vi "LoopselFF_1cam.VI"() -> ()   [LabVIEW 2015]
panel:
  out "Signalverlaufgraph":u16[](graph)=[0, 0, 0, 0, 0, 1, 0, 27665, 0, 0, 0, 0, 0, 0, 0, 0, 0, 0, 0, 0, 0, 0, 0, 0, 0, 0, 0, 0, 0, 0, 0, 0, 0, 0, 0, 0, 0, 0, 0, 0, 0, 0, 0, 0, 0, 0, 0, 0, 0, 0, 0, 0, 0, 0, 0, 0, 0, 0, 0, 0, 0, 0, 0, 0, 0, 0, 0, 0, 0, 0, 0, 0, 0, 0, 0, 0, 0, 0, 0, 0, 0, 0, 0, 0, 0, 0, 0, 0, 0, 0, 0, 0, 0, 0, 0, 0, 0, 0, 0, 0, 0, 0, 0, 0, 0, 0, 0, 0, 0, 0, 0, 0, 0, 0, 0, 0, 0, 0, 0, 0, 0, 0, 0, 0, 0, 0, 0, 0, 0, 0, 0, 0, 0, 0, 0, 0, 0, 0, 0, 0, 0, 0, 0, 0, 0, 0, 0, 0, 0, 0, 0, 0, 0, 0, 0, 0, 0, 0, 0, 0, 0, 0, 0, 0, 0, 0, 0, 0, 0, 0, 0, 0, 0, 0, 0, 0, 0, 0, 0, 0, 0, 0, 0, 0, 0, 0, 0, 0, 0, 0, 0, 0, 0, 0, 0, 0, 0, 0, 0, 0, 0, 0, 0, 0, 0, 0, 0, 0, 0, 0, 0, 0, 0, 0, 0, 0, 0, 0, 0, 0, 0, 0, 0, 0, 0, 0, 0, 0, 0, 0, 0, 0, 0, 0, 0, 0, 0, 0, 0, 0, 0, 0, 0, 0, 0, 0, 0, 0, 0, 0, 0, 0, 0, 0, 0, 0, 0, 0, 0, 0, 0, 0, 0, 0, 0, 0, 0, 0, 0, 0, 0, 0, 0, 0, 0, 0, 0, 0, 0, 0, 0, 0, 0, 0, 0, 0, 0, 0, 0, 0, 0, 0, 0, 0, 0, 0, 0, 0, 0, 0, 0, 0, 0, 0, 0, 0, 0, 0, 0, 0, 0, 0, 0, 0, 0, 0, 0, 0, 0, 0, 0, 0, 0, 0, 0, 0, 0, 0, 0, 0, 0, 0, 0, 0, 0, 0, 0, 0, 0, 0, 0, 0, 0, 0, 0, 0, 0, 0, 0, 0, 0, 0, 0, 0, 0, 0, 0, 0, 0, 0, 0, 0, 0, 0, 0, 0, 0, 0, 0, 0, 0, 0, 0, 0, 0, 0, 0, 0, 0, 0, 0, 0, 0, 0, 0, 0, 0, 0, 0, 0, 0, 0, 0, 0, 0, 0, 0, 0, 0, 0, 0, 0, 0, 0, 0, 0, 0, 0, 0, 0, 0, 0, 0, 0, 0, 0, 0, 0, 0, 0, 0, 0, 0, 0, 0, 0, 0, 0, 0, 0, 0, 0, 0, 0, 0, 0, 0, 0, 0, 0, 0, 0, 0, 0, 0, 0, 0, 0, 0, 0, 0, 0, 0, 0, 0, 0, 0, 0, 0, 0, 0, 0, 0, 0, 0, 0, 0, 0, 0, 0, 0, 0, 0, 0, 0, 0, 0, 0, 0, 0, 0, 0, 0, 0, 0, 0, 0, 0, 0, 0, 0, 0, 0, 0, 0, 0, 0, 0, 0, 0, 0, 0, 0, 0, 0, 0, 0, 0, 0, 0, 0, 0, 0, 0, 0, 0, 0, 0, 0, 0, 0, 0, 0, 0, 0, 0, 0, 0, 0, 0, 0, 0, 0, 0, 0, 0, 0, 0, 0, 0, 0, 0, 0, 0, 0, 0, 0, 0, 0, 0, 0, 0, 0, 0, 0, 0, 0, 0, 0, 0, 0, 0, 0, 0, 0, 0, 0, 0, 0, 0, 0, 0, 0, 0, 0, 0, 0, 0, 0, 0, 0, 0, 0, 0, 0, 0, 0, 0, 0, 0, 0, 0, 0, 0, 0, 0, 0, 0, 0, 0, 0, 0, 0, 0, 0, 0, 0, 0, 0, 0, 0, 0, 0, 0, 0, 0, 0, 0, 0, 0, 0, 0, 0, 0, 0, 0, 0, 0, 0, 0, 0, 0, 0, 0, 0, 0, 0, 0, 0, 0, 0, 0, 0, 0, 0, 0, 0, 0, 0, 0, 0, 0, 0, 0, 0, 0, 0, 0, 0, 0, 0, 0, 0, 0, 0, 0, 0, 0, 0, 0, 0, 0, 0, 0, 0, 0, 0, 0, 0, 0, 0, 0, 0, 0, 0, 0, 0, 0, 0, 0, 0, 0, 0, 0, 0, 0, 0, 0, 0, 0, 0, 0, 0, 0, 0, 0, 0, 0, 0, 0, 0, 0, 0, 0, 0, 0, 0, 0, 0, 0, 0, 0, 0, 0, 0, 0, 0, 0, 0, 0, 0, 0, 0, 0, 0, 0, 0, 0, 0, 0, 0, 0, 0, 0, 0, 0, 0, 0, 0, 0, 0, 0, 0, 0, 0, 0, 0, 0, 0, 0, 0, 0, 0, 0, 0, 0, 0, 0, 0, 0, 0, 0, 0, 0, 0, 0, 0, 0, 0, 0, 0, 0, 0, 0, 0, 0, 0, 0, 0, 0, 0, 0, 0, 0, 0, 0, 0, 0, 0, 0, 0, 0, 0, 0, 0, 0, 0, 0, 0, 0, 0, 0, 0, 0, 0, 0, 0, 0, 0, 0, 0, 0, 0, 0, 0, 0, 0, 0, 0, 0, 0, 0, 0, 0, 0, 0, 0, 0, 0, 0, 0, 0, 0, 0, 0, 0, 0, 0, 0, 0, 0, 0, 0, 0, 0, 0, 0, 0, 0, 0, 0, 0, 0, 0, 0, 0, 0, 0, 0, 0, 0, 0, 0, 0, 0, 0, 0, 0, 0, 0, 0, 0, 0, 0, 0, 0, 0, 0, 0, 0, 0, 0, 0, 0, 0, 0, 0, 0, 0, 0, 0, 0, 0, 0, 0, 0, 0, 0, 0, 0, 0, 0, 0, 0, 0, 0, 0, 0, 0, 0, 0, 0, 0, 0, 0, 0, 0, 0, 0, 0, 0, 0, 0, 0, 0, 0, 0, 0, 0, 0, 0, 0, 0, 0, 0, 0, 0, 0, 0, 0, 0, 0, 0, 0, 0, 0, 0, 0, 0, 0, 0, 0, 0, 0, 0, 0, 0, 0, 0, 0, 0, 0, 0, 0, 0, 0, 0, 0, 0, 0, 0, 0, 0, 0, 0, 0, 0, 0, 0, 0, 0, 0, 0, 0, 0, 0, 0, 0, 0, 0, 0, 0, 0, 0, 0, 0, 0, 0, 0, 0, 0, 0, 0, 0, 0, 0, 0, 0, 0, 0, 0, 0, 0, 0, 0, 0, 0, 0, 0, 0, 0, 0, 0, 0, 0, 0, 0, 0, 0, 0, 0, 0, 0, 0, 0, 0, 0, 0, 0, 0, 0, 0, 0, 0, 0, 0, 0, 0, 0, 0, 0, 0, 0, 0, 0, 0, 0, 0, 0, 0, 0, 0, 0, 0, 0, 0, 0, 0, 0, 0, 0, 0, 0, 0, 0, 0, 0, 0]
  in  "Slide":u32(slide)=27666 scale=1.0..60000.0
  in  "stop all":bool
  out "FIFO overflow 2":bool
  in  "extTrig 0/1":u8
  in  "frequency[Hz]":u32
  in  "start new block":bool
  in  "alloc mem":bool
  out "FREE \nRAM MB":u64=14179
  out "BUILT-IN\nRAM MB":u64=16662
  out "SEC":dbl=1.2
  out "MB RAM":u64=125
  in  "pos slope":u8=1
  in  "both slopes":u8
  in  "DAT in 10ns":u32
  in  "no.of samples (nos)":u32=60000
  in  "exposuretime[ms]":dbl=0.02 format="%.3f"
  # "Start with run"
  # "Abort with ESC"
  # "1x"
  # "repeat"
  # "exit here"
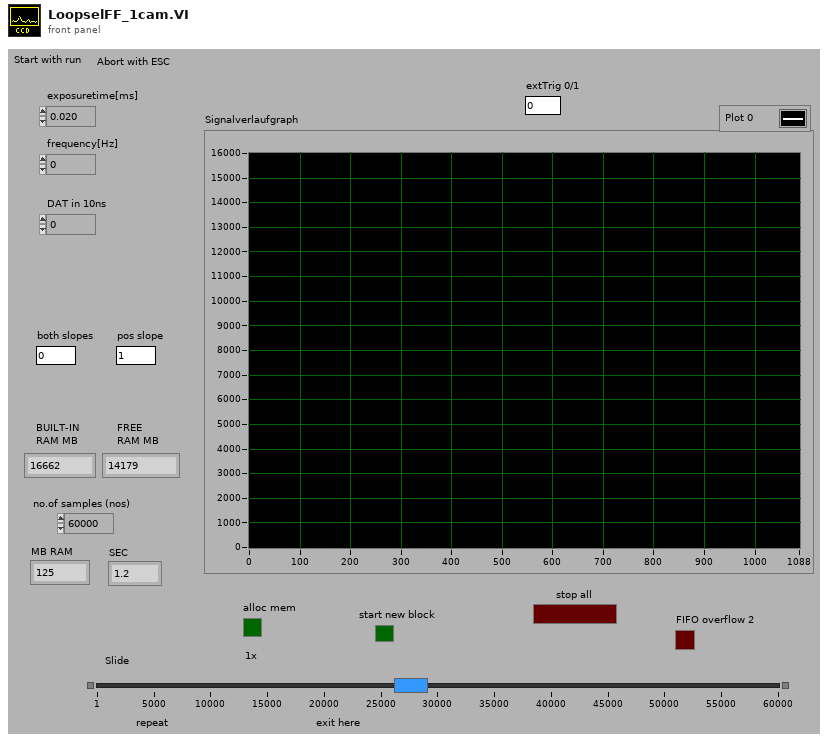
[diagram p1: front panel]
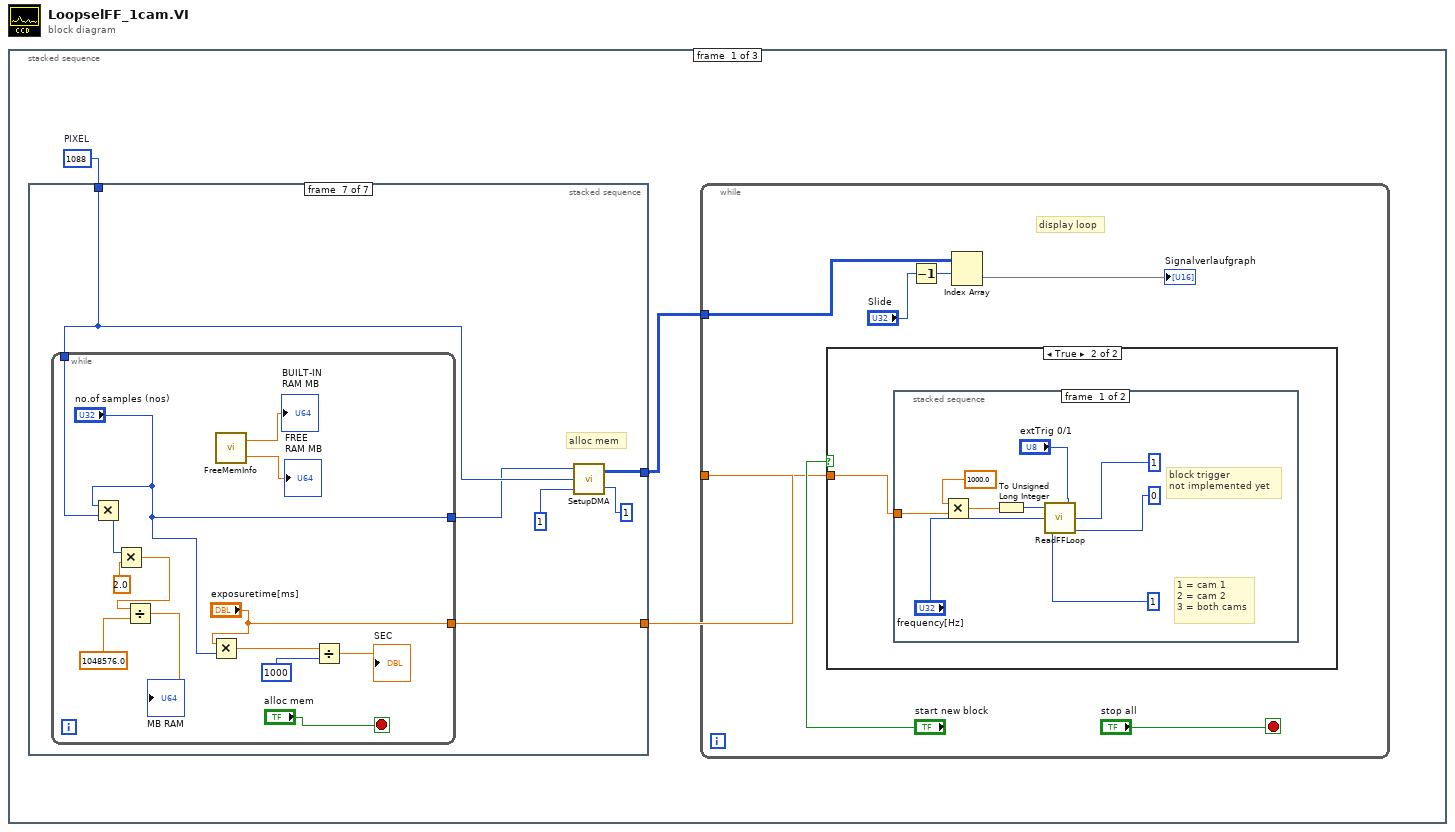
[diagram p0: block diagram]
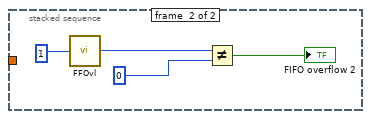
[diagram p3: hidden frame]
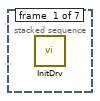
[diagram p4: hidden frame]
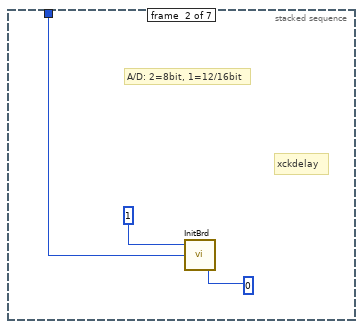
[diagram p5: hidden frame]
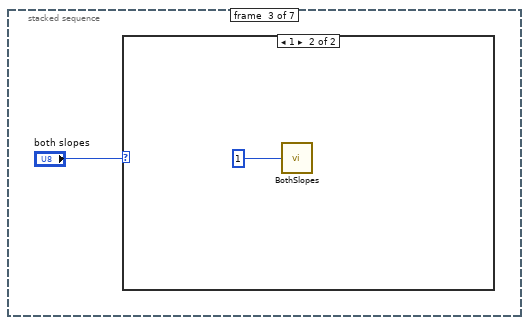
[diagram p6: hidden frame]
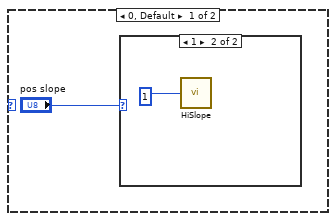
[diagram p7: hidden frame]
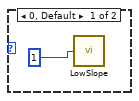
[diagram p8: hidden frame]
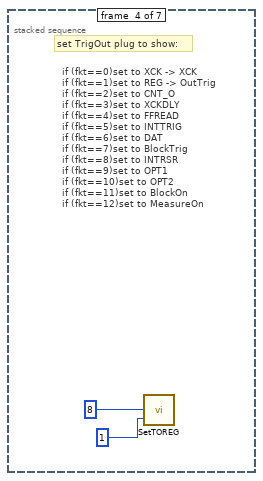
[diagram p9: hidden frame]
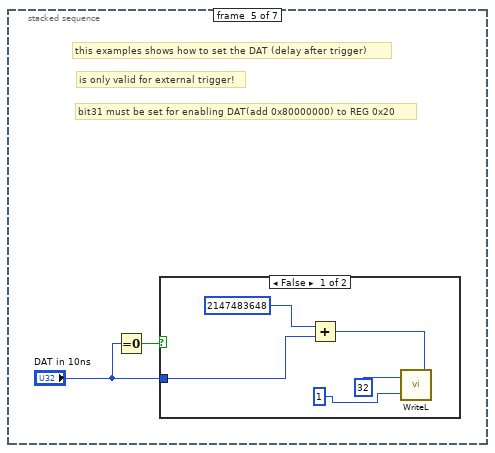
[diagram p10: hidden frame]
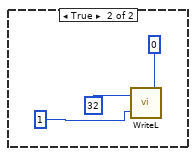
[diagram p11: hidden frame]
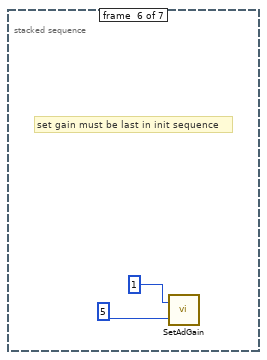
[diagram p12: hidden frame]
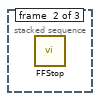
[diagram p13: hidden frame]
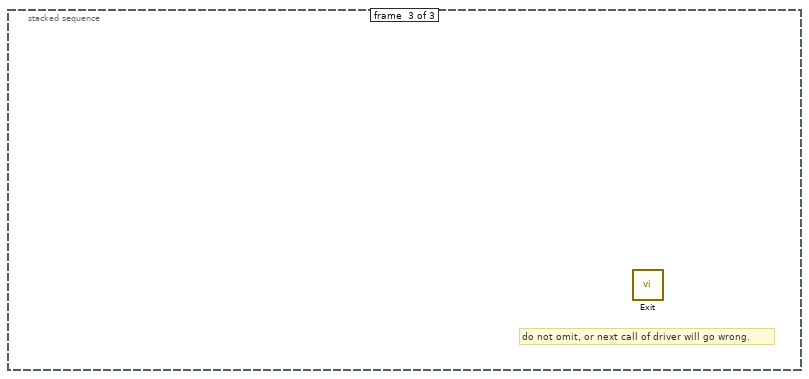
[diagram p14: hidden frame]
diagram:
  n1 = stacked-sequence {
    frame #0 {
      w3 = u32 1088  # PIXEL
      n2 = stacked-sequence {
        tunnel: [_ _ _ _ _ _ w52] -> w1
        tunnel: [_ _ _ _ _ _ w50] -> w2
        tunnel: w3 -> [_ w25 _ _ _ _ w48]
        frame #0 {
          n3 = call "InitDrv.vi"() -> ()  [unwired: 1 in, 1 out]
        }
        frame #1 {
          # "xckdelay"
          # "A/D: 2=8bit, 1=12/16bit"
          n4 = call "InitBrd.vi"("xckdly"=u32 0, "pixel"=w25, "flag816"=u32 1) -> ()  [unwired: 3 in]
        }
        frame #2 {
          n5 = case shown="1" "both slopes" {
            frame 0, Default {
              n6 = case shown="1" "pos slope" {
                frame 0, Default {
                  n7 = call "LowSlope.vi"("board"=1) -> ()  [unwired: 1 in]
                }
                frame 1 {
                  n8 = call "HiSlope.vi"("board"=1) -> ()  [unwired: 1 in]
                }
              }
            }
            frame 1 {
              n9 = call "BothSlopes.vi"("board"=1) -> ()  [unwired: 1 in]
            }
          }
        }
        frame #3 {
          # "set TrigOut plug to show:"
          # "if (fkt==0)set to XCK -> XCK\nif (fkt==1)set to REG -> OutTrig\nif (fkt==2)set to CNT_O\nif (fkt==3)set to XCKDLY\nif (fkt==4)set to FFREAD\nif (fkt==5)set to INTTRIG\nif (fkt==6)set to DAT\nif (fkt==7)set to BlockTrig\nif (fkt==8)set to INTRSR\nif (fkt==9)set to OPT1\nif (fkt==10)set to OPT2\nif (fkt==11)set to BlockOn\nif (fkt==12)set to MeasureOn"
          n10 = call "SetTOREG.vi"("board"=1, "fkt"=u8 8) -> ()  [unwired: 1 in]
        }
        frame #4 {
          # "bit31 must be set for enabling DAT(add 0x80000000) to REG 0x20"
          # "is only valid for external trigger!"
          # "this examples shows how to set the DAT (delay after trigger)"
          n11 = Equal To 0?(x="DAT in 10ns") -> (x = 0?=w36:bool)
          n12 = case shown="False" w36 {
            tunnel: "DAT in 10ns" -> [w38 _]
            frame False {
              n13 = Add(x=u32 2147483648, y=w38) -> (x+y=w41:u32)
              n14 = call "WriteL.vi"("val"=w41, "board"=1, "offset"=u32 32) -> ()
            }
            frame True {
              n15 = call "WriteL.vi"("val"=0, "board"=1, "offset"=u32 32) -> ()
            }
          }
        }
        frame #5 {
          # "set gain must be last in init sequence"
          n16 = call "SetAdGain.vi"("gain"=u8 5, "board"=1) -> ()  [unwired: 1 in]
        }
        frame #6 {
          # "alloc mem"
          n17 = while {
            tunnel: w48 -> [w62]
            tunnel: ["exposuretime[ms]"] -> w50
            tunnel: ["no.of samples (nos)"] -> w47
            stop <- "alloc mem" stop-if-true
            n18 = Multiply(x="no.of samples (nos)", y=w62) -> (x*y=w63:u32)
            n19 = Multiply(x=w63, y=2.0) -> (x*y=w64:dbl)
            n20 = Divide(x=w64, y=1048576.0) -> (x/y=→"MB RAM":dbl)
            n21 = Multiply(x="exposuretime[ms]", y="no.of samples (nos)") -> (x*y=w59:dbl)
            n22 = call "FreeMemInfo.vi"() -> ("PhysicalSpace"=→"BUILT-IN\nRAM MB":dbl, "PhysicalFreeSpace"=→"FREE \nRAM MB":dbl)  [unwired: 1 in]
            n23 = Divide(x=w59, y=1000) -> (x/y=→"SEC":dbl)
          }
          n24 = call "SetupDMA.vi"("blocks"=1, "Drv"=1, "pixel"=w48, "nos"=w47) -> ("Data Values"=w52:u16[][])
        }
      }
      n25 = while {
        tunnel: w1 -> [w10]
        tunnel: w2 -> [w5]
        stop <- "stop all" stop-if-true
        # "display loop"
        n26 = case shown="True" "start new block" {
          tunnel: w5 -> [_ w11]
          frame False {
          }
          frame True {
            n27 = stacked-sequence {
              tunnel: w11 -> [w12 _]
              frame #0 {
                # "1 = cam 1\n2 = cam 2\n3 = both cams"
                # "block trigger \nnot implemented yet"
                n28 = Multiply(x=1000.0, y=w12) -> (x*y=w18:dbl)
                n29 = To Unsigned Long Integer(number=w18) -> (unsigned 32bit integer=w14:u32)
                n30 = call "ReadFFLoop.vi"("blocktrigger"=u8 0, "btrig_ch"=u8 1, "ExtTrig"="extTrig 0/1", "cam_sel"=u8 1, "freq"="frequency[Hz]", "exptus"=w14) -> ()
              }
              frame #1 {
                n31 = call "FFOvl.vi"("Drv"=1) -> ("FFOvl"=w23:u8)
                n32 = Not Equal?(x=w23, y=0) -> (x != y?=→"FIFO overflow 2":bool)
              }
            }
          }
        }
        n33 = Decrement(x="Slide") -> (x-1=w7:u32)
        n34 = Index Array(array=w10, index (row)=w7) -> (element=→"Signalverlaufgraph":u16[])  [unwired: 1 in]
      }
    }
    frame #1 {
      n35 = call "FFStop.vi"() -> ()  [unwired: 1 in]
    }
    frame #2 {
      # "do not omit, or next call of driver will go wrong."
      n36 = call "Exit.vi"() -> ()  [unwired: 1 in]
    }
  }
